vi "Are Equal.vi"(8 "error in":errorcluster, 9 "Received Text":string, 10 "Approved Text":string, 11 "Text Comparator in":refnum<class "Text Comparator.lvclass">) -> (0 "error out":errorcluster, 2 "Are Equal?":bool, 3 "Text Comparator out":refnum<class "Text Comparator.lvclass">)   [LabVIEW 2020, in "Approval Tests.lvlib" / "Text Comparator.lvclass"]
uses:
  Text Comparator.lvclass
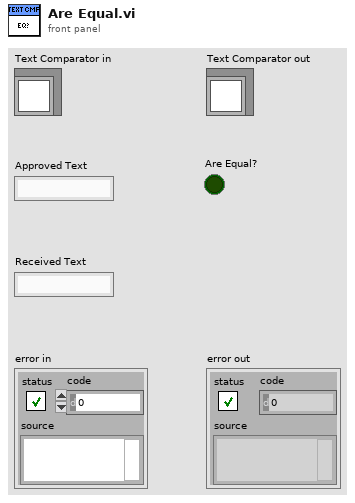
[diagram p1: front panel]
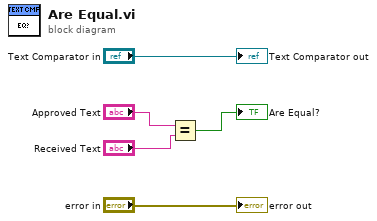
[diagram p0: block diagram]
diagram:
  n1 = Equal?(x="Approved Text", y="Received Text") -> (x = y?=→"Are Equal?":bool)
  "error out" <- "error in"
  "Text Comparator out" <- "Text Comparator in"
